vi "nxt main.vi"() -> ()   [LabVIEW 2012, in "Tugboat.lvrbt"]
uses:
  Tugboat.lvrbt
  tugProperties_t.ctl
  sensorData_t.ctl
  irData_t.ctl
  motorData_t.ctl
  motorCommands_t.ctl
  <vilib>/NXT/Block Support/NXT_TimerIndex.ctl
  behaviorWeights_t.ctl
panel:
  out "x+y":dbl
  in  "_sendToPC":string
  in  "_fromPC":u8[](array[numeric])
  out "Sense/Act":bool=TRUE
  in  "_motorCommands":T1={"_rudderCommand"=7, "_propCommand"=7, "_irServoCommand"=7}
  in  "_motorData":T2={"_rudderCommand"=1450, "_propCommand"=1500, "_irServoCommand"=1550}
  in  "_sensorData":T3
  in  "Tugboat Properties":T5={"_name"="Enterprise", "_pitch"=440, "_rudderCenter"=1450, "_propCenter"=1500, "_irServoCenter"=1550, "_rudderMin"=930, "_rudderMax"=2000, "_propMin"=1000, "_propMax"=2000, "_irServoMin"=800, "_irServoMax"=2200}
  in  "SOFT E-STOP":bool
  in  "HARD E-STOP":bool
  # "L\nE\nF\nT"
  # "C\nE\nN\nT\nE\nR"
  # "R\nI\nG\nH\nT"
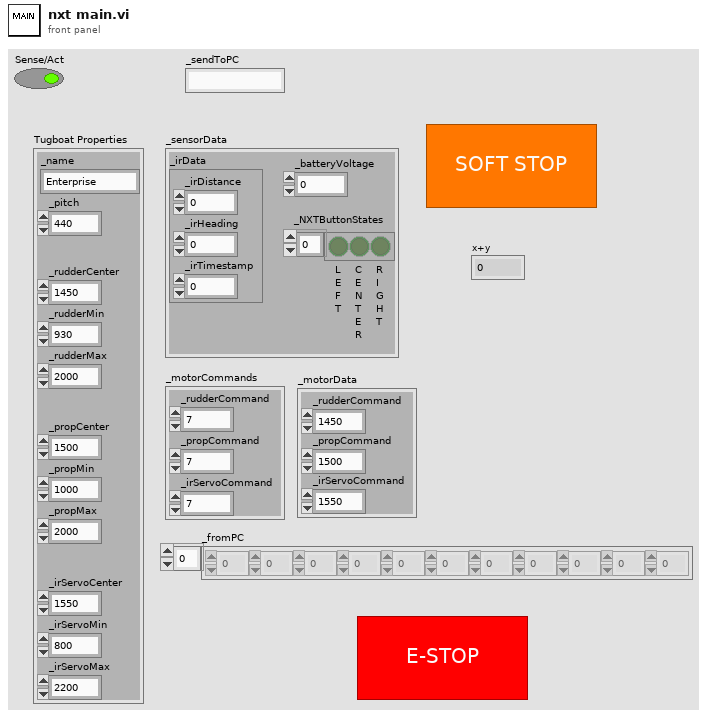
[diagram p1: front panel]
types:
  T1 = typedef "motorCommands_t.ctl" = cluster{"_rudderCommand":i8, "_propCommand":i8, "_irServoCommand":i8}
  T2 = typedef "motorData_t.ctl" = cluster{"_rudderCommand":u16, "_propCommand":u16, "_irServoCommand":u16}
  T3 = typedef "sensorData_t.ctl" = cluster{"_irData":T4, "_batteryVoltage":i32, "_NXTButtonStates":bool[]}
  T4 = typedef "irData_t.ctl" = cluster{"_irDistance":i32, "_irHeading":i32, "_irTimestamp":u32}
  T5 = typedef "tugProperties_t.ctl" = cluster{"_name":string, "_pitch":i32, "_rudderCenter":u16, "_propCenter":u16, "_irServoCenter":u16, "_rudderMin":u16, "_rudderMax":u16, "_propMin":u16, "_propMax":u16, "_irServoMin":u16, "_irServoMax":u16}
  T6 = typedef "behaviorWeights_t.ctl" = i8[]
  T7 = typedef "NXT_TimerIndex.ctl" = u8
  T8 = typedef "LVHSConnector.ctl" = cluster{"Hardware":string, "Flattened String":string}
  T9 = typedef "behaviorOutput_t.ctl" = cluster{"Goodness":i8[], "Velocity":i8[], "Weight":i8}
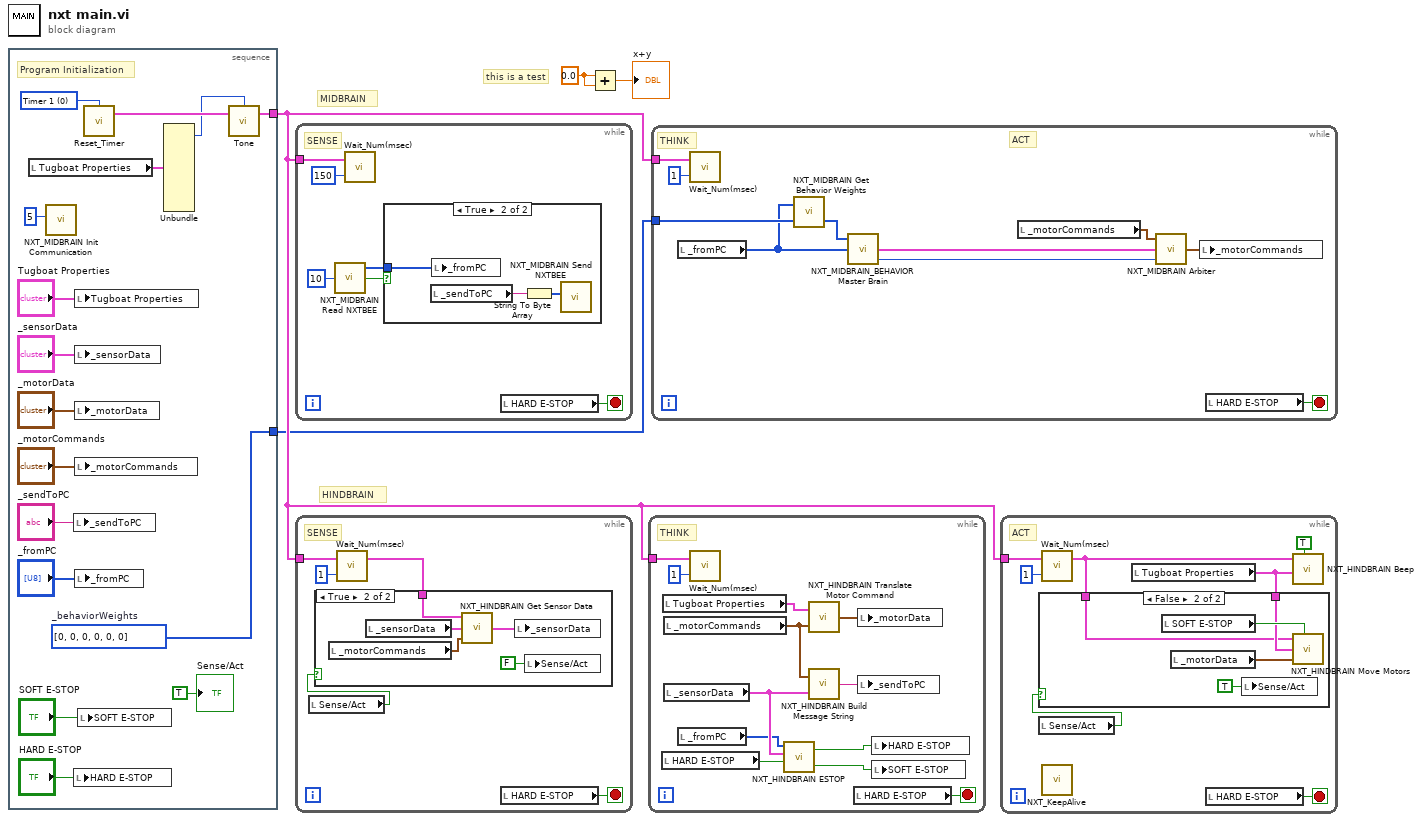
[diagram p0: block diagram]
diagram:
  w2 = 0.0 ("x")
  # "this is a test"
  # "HINDBRAIN"
  # "MIDBRAIN"
  n1 = stacked-sequence {
    tunnel: [w14] -> w4
    tunnel: [w8] -> w3
    frame #0 {
      w8 = T6 [0, 0, 0, 0, 0, 0]  # _behaviorWeights
      w16 = T7 0 items=["Timer 1", "Timer 2", "Timer 3"] ("Timer (Timer 1)")
      # "Program Initialization"
      n2 = local read "Tugboat Properties"() -> (w19:T5)
      n3 = call "NXT_MIDBRAIN Init Communication.vi"("Speed"=u8 5) -> ()  [unwired: 6 in, 1 out]
      n4 = local write "_sendToPC"("_sendToPC") -> ()
      n5 = local write "HARD E-STOP"("HARD E-STOP") -> ()
      n6 = local write "Tugboat Properties"("Tugboat Properties") -> ()
      n7 = local write "_sensorData"("_sensorData") -> ()
      n8 = local write "_motorData"("_motorData") -> ()
      n9 = local write "_motorCommands"("_motorCommands") -> ()
      n10 = local write "_fromPC"("_fromPC") -> ()
      n11 = local write "SOFT E-STOP"("SOFT E-STOP") -> ()
      n12 = call <vilib>:"Reset_Timer.vi"("Timer (Timer 1)"=w16) -> ("NXT"=w11:T8)  [unwired: 3 in]
      n13 = Unbundle(w19) -> ("_pitch"=w9:i32)  [unwired: 10 out]
      n14 = call <vilib>:"Tone.vi"("NXT"=w11, "Tone (440 Hz)"=w9) -> ("NXT"=w14:T8)  [unwired: 2 in]
      "Sense/Act" <- TRUE ("Sense/Act")
    }
  }
  n15 = while {
    tunnel: w4 -> [w25]
    stop <- w24 stop-if-true
    # "SENSE"
    n16 = call "NXT_MIDBRAIN Read NXTBEE.vi"("#bytes"=u8 10) -> ("Valid String?"=w21:bool, "Data Out"=w23:u8[])  [unwired: 2 in, 1 out]
    n17 = call <vilib>:"Wait_Num(msec).vi"("Time (100 msec)"=u32 150, "NXT"=w25) -> ()  [unwired: 2 in, 1 out]
    n18 = case shown="True" w21 {
      tunnel: w23 -> [_ w27]
      frame False {
      }
      frame True {
        n19 = local read "_sendToPC"() -> (w28:string)
        n20 = local write "_fromPC"(w27) -> ()
        n21 = String To Byte Array(string=w28) -> (unsigned byte array=w29:u8[])
        n22 = call "NXT_MIDBRAIN Send NXTBEE.vi"("Data"=w29) -> ()  [unwired: 8 in, 1 out]
      }
    }
    n23 = local read "HARD E-STOP"() -> (w24:bool)
  }
  n24 = while {
    tunnel: w4 -> [w31]
    stop <- w33 stop-if-true
    # "SENSE"
    n25 = local read "Sense/Act"() -> (w30:bool)
    n26 = call <vilib>:"Wait_Num(msec).vi"("Time (100 msec)"=u32 1, "NXT"=w31) -> ("NXT"=w32:T8)  [unwired: 2 in]
    n27 = case shown="True" w30 {
      tunnel: w32 -> [_ w39]
      frame False {
      }
      frame True {
        n28 = local read "_motorCommands"() -> (w37:T1)
        n29 = local read "_sensorData"() -> (w38:T3)
        n30 = call "NXT_HINDBRAIN Get Sensor Data.vi"("_motorCommands"=w37, "_sensorData"=w38, "NXT"=w39) -> ("_sensorData"=w36:T3)  [unwired: 2 in]
        n31 = local write "_sensorData"(w36) -> ()
        n32 = local write "Sense/Act"(FALSE ("Sense/Act")) -> ()
      }
    }
    n33 = local read "HARD E-STOP"() -> (w33:bool)
  }
  n34 = Add(x=w2, y=w2) -> (x+y=→"x+y":dbl)
  n35 = while {
    tunnel: w4 -> [w49]
    stop <- w50 stop-if-true
    # "THINK"
    n36 = local read "HARD E-STOP"() -> (w41:bool)
    n37 = local read "Tugboat Properties"() -> (w47:T5)
    n38 = local read "_motorCommands"() -> (w45:T1)
    n39 = local read "_sensorData"() -> (w44:T3)
    n40 = local read "_fromPC"() -> (w43:u8[])
    n41 = call <vilib>:"Wait_Num(msec).vi"("Time (100 msec)"=u32 1, "NXT"=w49) -> ()  [unwired: 2 in, 1 out]
    n42 = call "NXT_HINDBRAIN ESTOP.vi"("Hard E-Stop"=w41, "_sensorData"=w44, "_fromPC"=w43) -> ("Soft E-Stop"=w42:bool, "Hard E-Stop"=w48:bool)  [unwired: 1 in]
    n43 = call "NXT_HINDBRAIN Translate Motor Command.vi"("_motorCommands"=w45, "Tugboat Properties"=w47) -> ("_motorData"=w46:T2)
    n44 = call "NXT_HINDBRAIN Build Message String.vi"("_sensorData"=w44, "_motorCommands"=w45) -> ("Data Out"=w40:string)
    n45 = local read "HARD E-STOP"() -> (w50:bool)
    n46 = local write "_motorData"(w46) -> ()
    n47 = local write "_sendToPC"(w40) -> ()
    n48 = local write "HARD E-STOP"(w48) -> ()
    n49 = local write "SOFT E-STOP"(w42) -> ()
  }
  n50 = while {
    tunnel: w4 -> [w61]
    tunnel: w3 -> [w60]
    stop <- w53 stop-if-true
    # "ACT"
    # "THINK"
    n51 = local read "_fromPC"() -> (w52:u8[])
    n52 = call <vilib>:"Wait_Num(msec).vi"("Time (100 msec)"=u32 1, "NXT"=w61) -> ()  [unwired: 2 in, 1 out]
    n53 = call "NXT_MIDBRAIN Get Behavior Weights.vi"("_behaviorWeights"=w60, "_fromPC"=w52) -> ("_behaviorWeights"=w58:T6)  [unwired: 1 in]
    n54 = call "NXT_MIDBRAIN_BEHAVIOR Master Brain.vi"("_fromPC"=w52, "_behaviorWeights"=w58) -> ("_irTheta"=w54:i8, "_behaviorData"=w55:T9[])  [unwired: 2 in]
    n55 = local read "_motorCommands"() -> (w57:T1)
    n56 = call "NXT_MIDBRAIN Arbiter.vi"("_irServoCommand"=w54, "Behavior Data"=w55, "_motorCommands"=w57) -> ("_motorCommands"=w56:T1)
    n57 = local write "_motorCommands"(w56) -> ()
    n58 = local read "HARD E-STOP"() -> (w53:bool)
  }
  n59 = while {
    tunnel: w4 -> [w65]
    stop <- w66 stop-if-true
    # "ACT"
    n60 = local read "Sense/Act"() -> (w62:bool)
    n61 = call <vilib>:"Wait_Num(msec).vi"("Time (100 msec)"=u32 1, "NXT"=w65) -> ("NXT"=w63:T8)  [unwired: 2 in]
    n62 = call <vilib>:"NXT_KeepAlive.vi"() -> ()  [unwired: 10 in, 2 out]
    n63 = local read "Tugboat Properties"() -> (w64:T5)
    n64 = case shown="False" w62 {
      tunnel: w64 -> [_ w72]
      tunnel: w63 -> [_ w70]
      frame True {
      }
      frame False {
        n65 = local read "SOFT E-STOP"() -> (w73:bool)
        n66 = local read "_motorData"() -> (w71:T2)
        n67 = local write "Sense/Act"(TRUE ("Sense/Act")) -> ()
        n68 = call "NXT_HINDBRAIN Move Motors.vi"("NXT"=w70, "Motor Disable"=w73, "Tugboat Properties"=w72, "_motorData"=w71) -> ()  [unwired: 2 in]
      }
    }
    n69 = local read "HARD E-STOP"() -> (w66:bool)
    n70 = call "NXT_HINDBRAIN Beep.vi"("NXT"=w63, "Beep Enable"=TRUE, "Tugboat Properties"=w64) -> ()  [unwired: 3 in]
  }
